vi "IV Programa 1_2.vi"() -> ()   [LabVIEW 2020]
panel:
  in  "Universal \nProgram STOP":bool
  out "String":string
  in  "String":string
  out "lts":dbl(slide) scale=0.0..10.0
  in  "lts":dbl(slide) scale=0.0..10.0
  out "?":bool
  in  "on/off":bool
  out "age":i32
  in  "age":i32
  # "1.2: Elabore un diagrama de bloques que contenga 1 control para cada uno de los tipos de datos básicos\n(INT, DBL, Boolean, String) y los deberá mostrar en un indicador."
  # "Numeric control to numeric indicator: \nInt"
  # "the slide control transmit\na value to a tank indicator.\n\nDBL"
  # "bolean switch (on off) on the left that controls on-off state\non the right light indicator. \n\nBolean"
  # "write in the left to see tha same in the right. \n\nString"
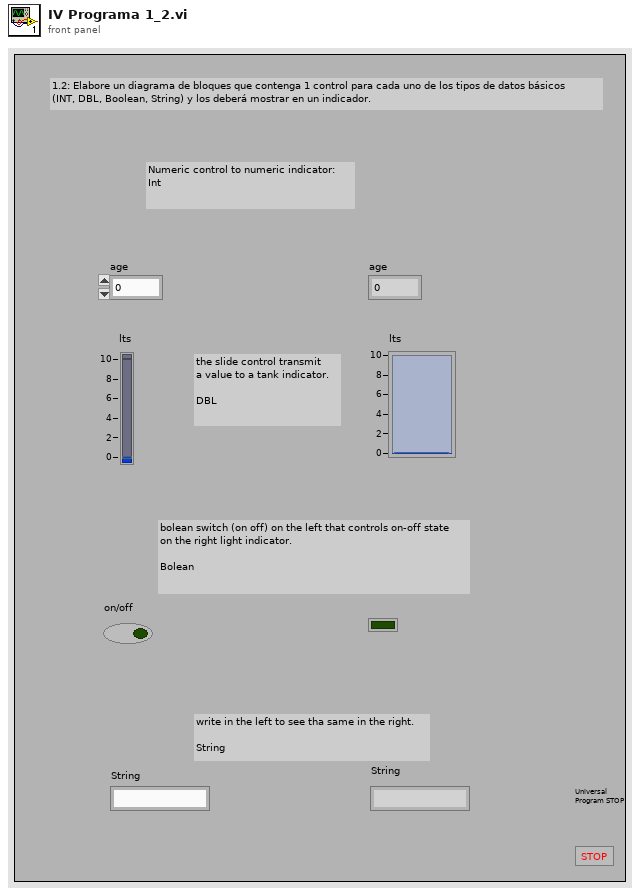
[diagram p1: front panel]
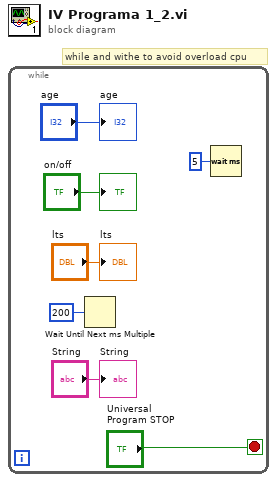
[diagram p0: block diagram]
diagram:
  # "while and withe to avoid overload cpu"
  n1 = while {
    stop <- "Universal \nProgram STOP" stop-if-true
    n2 = Wait Until Next ms Multiple(millisecond multiple=u32 200) -> ()  [unwired: 1 out]
    n3 = Wait (ms)(milliseconds to wait=u32 5) -> ()  [unwired: 1 out]
    "age" <- "age"
    "?" <- "on/off"
    "lts" <- "lts"
    "String" <- "String"
  }
